vi "GIC Builder 7.vi"(0 "Parameters":dbl[](array[numeric]), 1 "Use ?\nOff       On":bool[](array[boolean])=[TRUE, TRUE, FALSE, FALSE], 4 "Obst Lats and Longs":cluster{"Obst Lats":dbl[], "Obst Longs":dbl[]} {"Obst Longs" format="%#_8g"; "Obst Lats" format="%#_8g"}, 5 "Num of WPs":i16, 6 "Prop Com Port":refnum<visa-resource-name>, 7 "Real":bool, 8 "Compass Com Port":refnum<visa-resource-name>, 9 "GPS Com Port":refnum<visa-resource-name>, 10 "GPS Time interval":dbl=2.4, 11 "WP Lats and Longs":cluster{"WP Lats":dbl[], "WP Longs":dbl[]}) -> (3 "GIC Output":T2={"Real/Sim"=FALSE, "WP Lats and Longs"={"WP Lats"=[], "WP Longs"=[]}, "GPS Time Int"=0.0, "GPS Com Port"="", "Compass Com Port"="", "Prop Com Port"="", "GPS Data"=[], "Compass"=0.0, "LMS Vector"=[], "Vision Vector"=[], "Direction Cmd"=0.0, "Speed Cmd"=0.0, "Time of Last GPS"=0.0, "WP Vector"=[], "WP Number"=0, "Num of WPs"=0, "SW Map"=[], "Obst Lats and Longs"={"Obst Lats"=[], "Obst Longs"=[]}, "Parameters"=[], "Cluster"={"Path x nodes"=[], "Path y nodes"=[]}, "     Use ?\nOff       On"=[TRUE, TRUE, FALSE, FALSE]} {"Obst Lats and Longs"."Obst Longs" format="%#_8g"; "Obst Lats and Longs"."Obst Lats" format="%#_8g"})   [LabVIEW 2014]
panel:
  out "?":bool[](array[boolean])
  in  "Path Cluster":T1
  in  "WP Number":i32
  in  "WP Vector":dbl[](array[numeric])
  in  "Time of last GPS":dbl
  in  "Speed Cmd":dbl
  in  "Direction Cmd":dbl
  in  "Vision Vector":dbl[](array[numeric])
  in  "GPS Data":dbl[](array[numeric])
  # "GIC Builder"
  # "Comm Ports"
  # "Modes"
  # "Sim"
  # "Initial Data for Global Information Cluster"
  # "GPS"
  # "LMS"
  # "Vision"
  # "Prop"
  # "GPS"
  # "LMS"
  # "Vision"
  # "Prop"
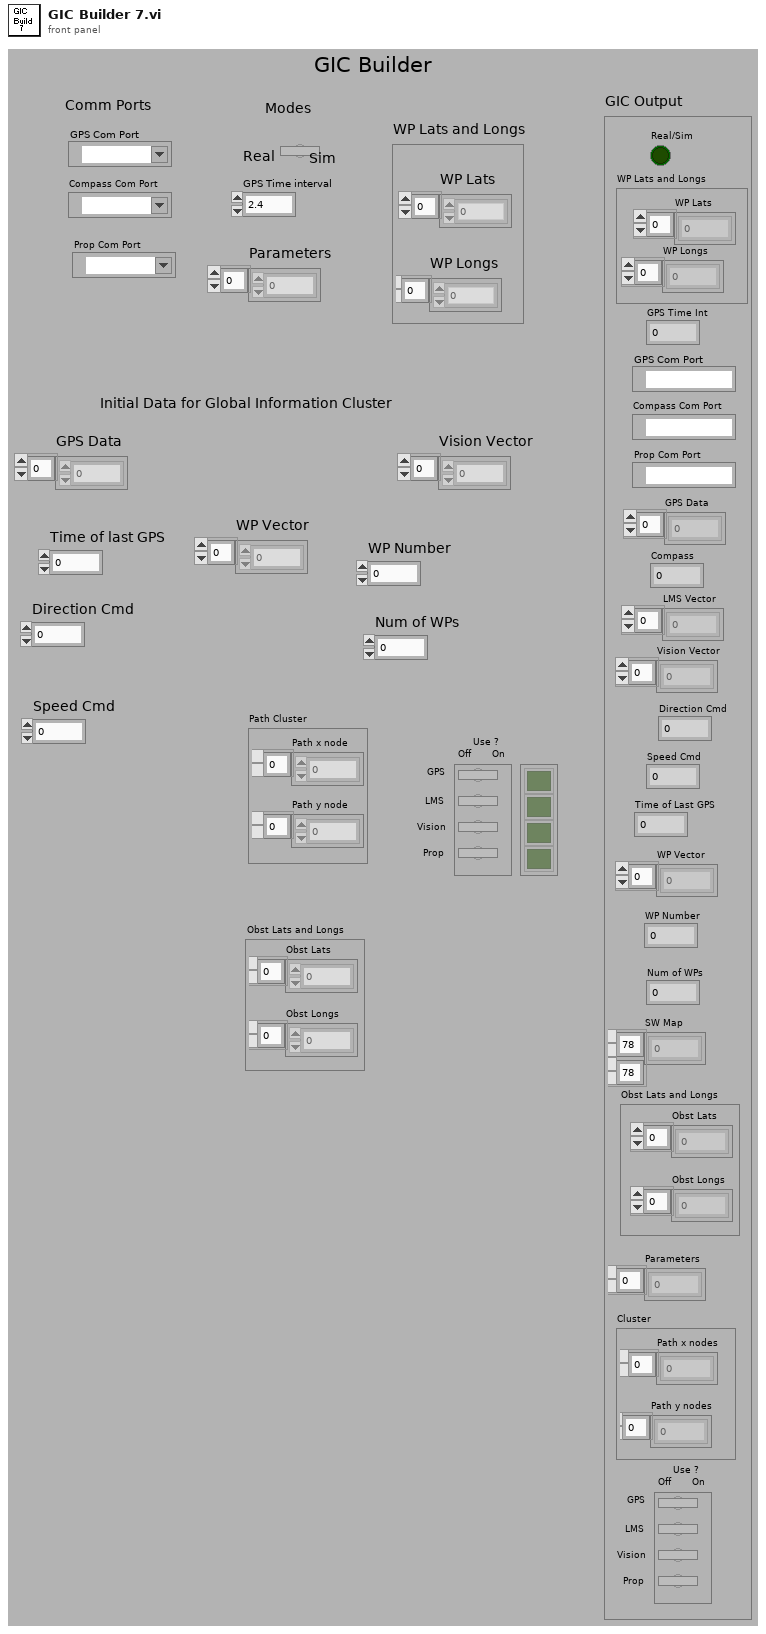
[diagram p1: front panel]
types:
  T1 = cluster{"Path x node":dbl[], "Path y node":dbl[]}
  T2 = cluster{"Real/Sim":bool, "WP Lats and Longs":cluster{"WP Lats":dbl[], "WP Longs":dbl[]}, "GPS Time Int":dbl, "GPS Com Port":refnum<visa-resource-name>, "Compass Com Port":refnum<visa-resource-name>, "Prop Com Port":refnum<visa-resource-name>, "GPS Data":dbl[], "Compass":dbl, "LMS Vector":dbl[], "Vision Vector":dbl[], "Direction Cmd":dbl, "Speed Cmd":dbl, "Time of Last GPS":dbl, "WP Vector":dbl[], "WP Number":i32, "Num of WPs":i16, "SW Map":i32[][], "Obst Lats and Longs":cluster{"Obst Lats":dbl[], "Obst Longs":dbl[]}, "Parameters":dbl[], "Cluster":cluster{"Path x nodes":dbl[], "Path y nodes":dbl[]}, "     Use ?\nOff       On":bool[]}
  T3 = cluster{"Real":bool, "WP Lats and Longs":cluster{"WP Lats":dbl[], "WP Longs":dbl[]}, "GPS Time interval":dbl, "GPS Com Port":refnum<visa-resource-name>, "Compass Com Port":refnum<visa-resource-name>, "Prop Com Port":refnum<visa-resource-name>, dbl[], "Numeric":dbl, dbl[], "Vision Vector":dbl[], "Direction Cmd":dbl, "Speed Cmd":dbl, "Time of last GPS":dbl, "WP Vector":dbl[], "WP Number":i32, "Num of WPs":i16, dbl[][], "Obst Lats and Longs":cluster{"Obst Lats":dbl[], "Obst Longs":dbl[]}, "Parameters":dbl[], "Path Cluster":cluster{"Path x node":dbl[], "Path y node":dbl[]}, "     Use ?\nOff       On":bool[]}
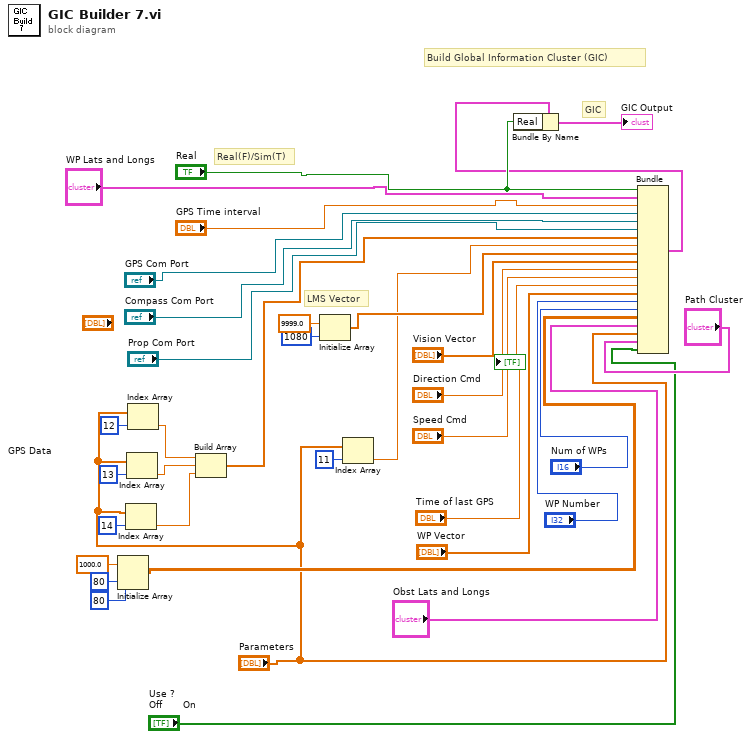
[diagram p0: block diagram]
diagram:
  # "LMS Vector"
  # "Real(F)/Sim(T)"
  # "GIC"
  # "Build Global Information Cluster (GIC)"
  n1 = Initialize Array(1000.0 ("element"), 80 ("dimension size"), 80 ("dimension size")) -> (w19:dbl[][])
  n2 = Index Array(array="Parameters", index=14) -> (element=w6:dbl)
  n3 = Index Array(array="Parameters", index=13) -> (element=w7:dbl)
  n4 = Index Array(array="Parameters", index=12) -> (element=w8:dbl)
  n5 = Build Array(w8, w7, w6) -> (w5:dbl[])
  n6 = Initialize Array(9999.0 ("element"), 1080 ("dimension size")) -> (w16:dbl[])
  n7 = Index Array(array="Parameters", index=11) -> (element=w13:dbl)
  n8 = Bundle("Real"="Real", "WP Lats and Longs"="WP Lats and Longs", "GPS Time interval"="GPS Time interval", "GPS Com Port"="GPS Com Port", "Compass Com Port"="Compass Com Port", "Prop Com Port"="Prop Com Port", w5, "Numeric"=w13, w16, "Vision Vector"="Vision Vector", "Direction Cmd"="Direction Cmd", "Speed Cmd"="Speed Cmd", "Time of last GPS"="Time of last GPS", "WP Vector"="WP Vector", "WP Number"="WP Number", "Num of WPs"="Num of WPs", w19, "Obst Lats and Longs"="Obst Lats and Longs", "Parameters"="Parameters", "Path Cluster"="Path Cluster", "Use ?\nOff       On"="Use ?\nOff       On") -> (w27:T3)  [unwired: 1 in]
  n9 = Bundle By Name(cluster=w27, "Real"="Real") -> (→"GIC Output":T3)
